vi "Splash Dequeue Command.vi"(8 "error in (no error)":errorcluster, 11 "Splash Queue in":refnum<queue>) -> (0 "error out":errorcluster, 1 "Message":string, 2 "Command":string, 3 "Splash Queue out":refnum<queue>)   [LabVIEW 2013, in "SET_Splash.lvlib"]
uses:
  SET_Splash.lvlib
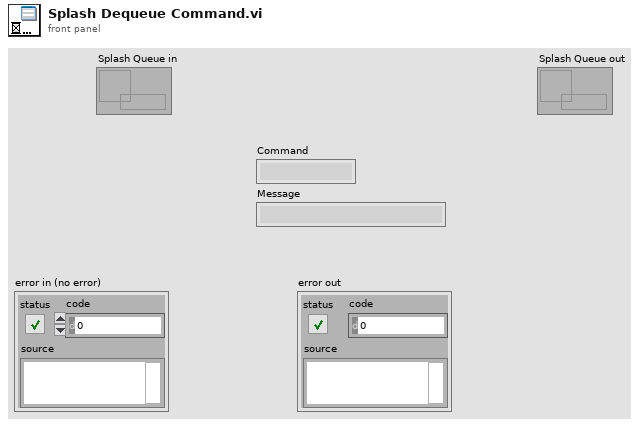
[diagram p1: front panel]
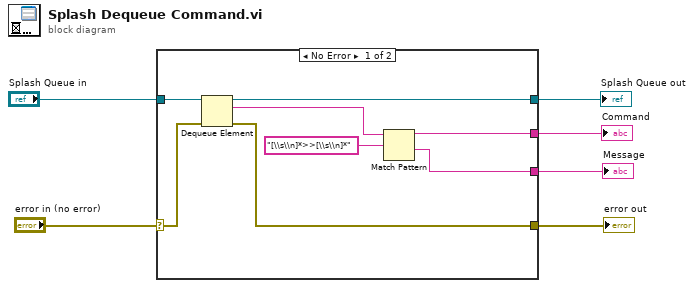
[diagram p0: block diagram]
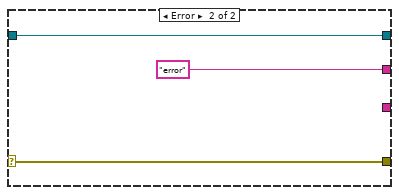
[diagram p2: hidden frame]
diagram:
  n1 = case shown="No Error" "error in (no error)" {
    selector: "error in (no error)" -> [w10 w17]
    tunnel: [w13 "error"] -> w6
    tunnel: [w12 _] -> w5
    tunnel: "Splash Queue in" -> [w8 w16]
    tunnel: [w7 w16] -> w1
    tunnel: [w9 w17] -> w3
    frame No Error {
      n2 = Dequeue Element(queue=w8, error in (no error)=w10) -> (queue out=w7:refnum<queue>, element=w11:string, error out=w9:errorcluster)  [unwired: 1 in, 1 out]
      n3 = Match Pattern(string=w11, regular expression="[\\s\\n]*>>[\\s\\n]*" ("search string/char (-)")) -> (before substring=w13:string, after substring=w12:string)  [unwired: 1 in, 2 out]
    }
    frame Error {
    }
  }
  "Command" <- w6
  "Message" <- w5
  "error out" <- w3
  "Splash Queue out" <- w1
